vi "Histogram Bin Size Definition Dialog.vi"(8 "error in (no error)":errorcluster, 9 "Dialog? (T)":bool=TRUE, 11 "Histogram Options in":T1={"Bin Size"=nan, "Min Value"=nan, "Max Value"=nan, "Filter NaN & Infinite Values"=FALSE, "Frequency Plot"=FALSE, "Align Bins"=FALSE, "Bin Location"=enum."Left", "Project Outside Values"=FALSE, "Max Histogram Size"=-1} {"Max Histogram Size" format="%.0e"}) -> (0 "error out":errorcluster, 1 "Cancelled?":bool, 3 "Histogram Options":T1={"Bin Size"=1.0, "Min Value"=1.0, "Max Value"=1.0, "Filter NaN & Infinite Values"=FALSE, "Frequency Plot"=FALSE, "Align Bins"=FALSE, "Bin Location"=enum."Left", "Project Outside Values"=FALSE, "Max Histogram Size"=1} {"Max Histogram Size" format="%.0e"})   [LabVIEW 2019, in "Histogram Window.lvlib"]
doc: "Displays a standard dialog box that prompts users to enter information, such as a user name and password.\n--------------------\n\nThis Express VI is configured as follows:\n\nMessage to Display to the User:Histogram bin to use:\nThe inputs are: \nNumber: Bin"
uses:
  Histogram Window.lvlib
  Linear Histogram Options.ctl
  Histogram Bin Position.ctl
panel:
  in  "Histogram Options":T1={"Bin Size"=nan, "Min Value"=-inf, "Max Value"=inf, "Filter NaN & Infinite Values"=TRUE, "Frequency Plot"=FALSE, "Align Bins"=FALSE, "Bin Location"=enum."Left", "Project Outside Values"=FALSE, "Max Histogram Size"=100000} {"Max Histogram Size" format="%.0e"}
  in  "Cancel":bool
  in  "OK":bool caption="OK1"
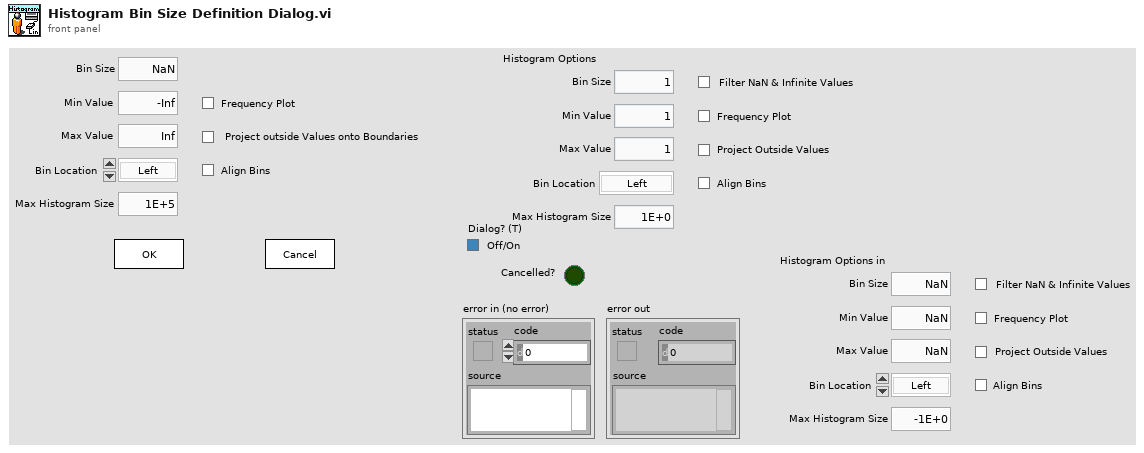
[diagram p1: front panel]
types:
  T1 = typedef "Linear Histogram Options.ctl" = cluster{"Bin Size":dbl, "Min Value":dbl, "Max Value":dbl, "Filter NaN & Infinite Values":bool, "Frequency Plot":bool, "Align Bins":bool, "Bin Location":T2, "Project Outside Values":bool, "Max Histogram Size":i32}
  T2 = typedef "Histogram Bin Position.ctl" = enum16{"Left", "Center", "Right"}
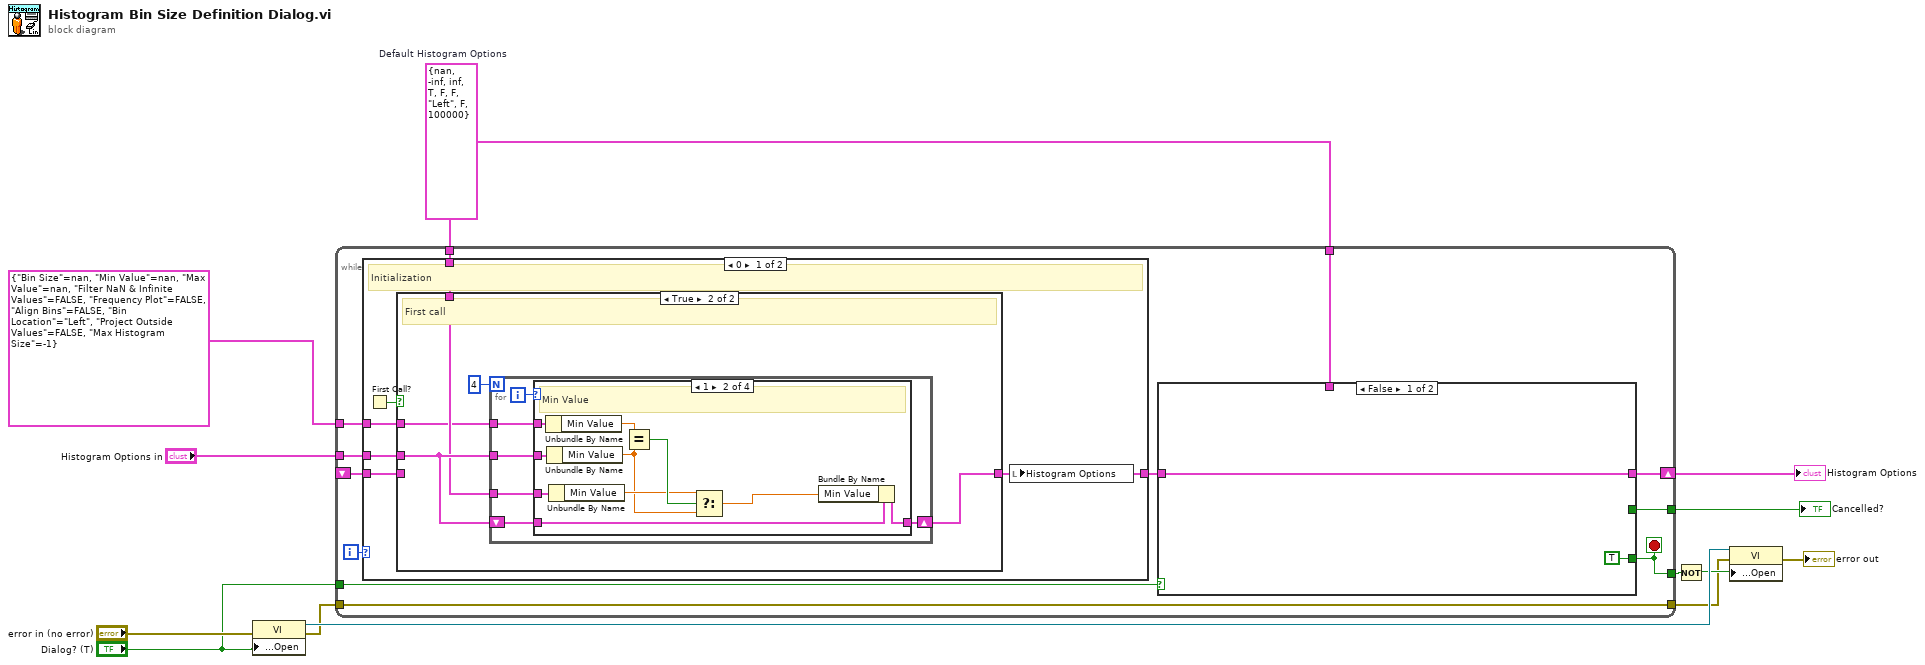
[diagram p0: block diagram]
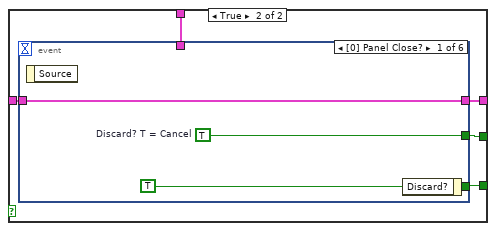
[diagram p2: hidden frame]
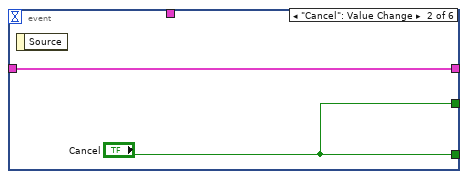
[diagram p3: hidden frame]
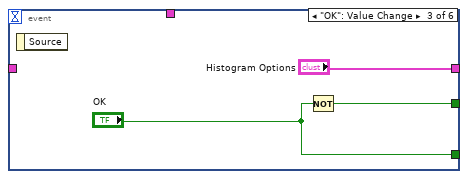
[diagram p4: hidden frame]
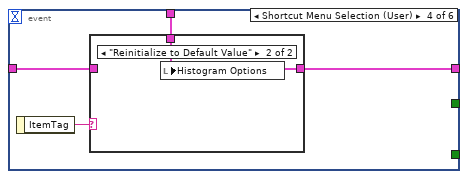
[diagram p5: hidden frame]
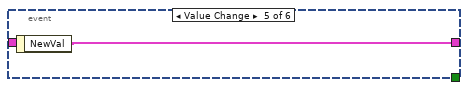
[diagram p7: hidden frame]
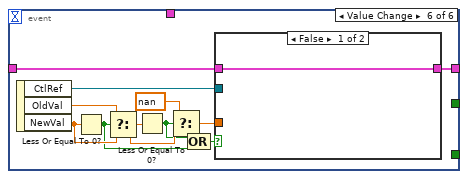
[diagram p8: hidden frame]
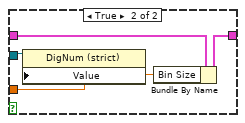
[diagram p9: hidden frame]
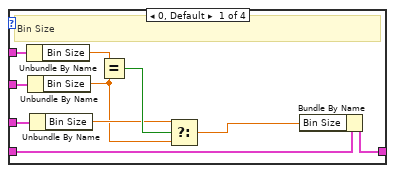
[diagram p11: hidden frame]
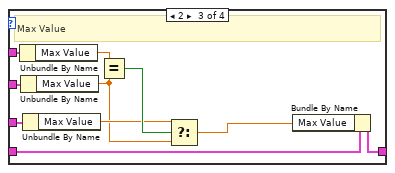
[diagram p12: hidden frame]
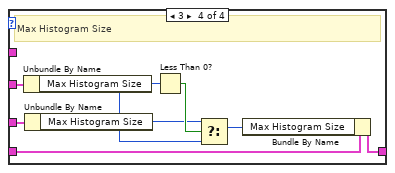
[diagram p13: hidden frame]
diagram:
  w6 = T1 {"Bin Size"=nan, "Min Value"=-inf, "Max Value"=inf, "Filter NaN & Infinite Values"=TRUE, "Frequency Plot"=FALSE, "Align Bins"=FALSE, "Bin Location"=enum."Left", "Project Outside Values"=FALSE, "Max Histogram Size"=100000}  # Default Histogram Options
  n1 = property class="VI"(error in="error in (no error)", "Front Panel Window:Open"="Dialog? (T)") -> (reference out=w10:refnum<vi>, error out=w5:errorcluster)  [unwired: 1 in]
  n2 = while {
    tunnel: [w25] -> w11
    tunnel: [w24] -> w9
    shift-right: [w23] -> w7
    shift-left: _ -> [w21]
    tunnel: w6 -> [w19]
    tunnel: w6 -> [w18]
    tunnel: "Histogram Options in" -> [w17]
    tunnel: w5 -> [w16]
    tunnel: [w16] -> w4
    tunnel: T1 {"Bin Size"=nan, "Min Value"=nan, "Max Value"=nan, "Filter NaN & Infinite Values"=FALSE, "Frequency Plot"=FALSE, "Align Bins"=FALSE, "Bin Location"=enum."Left", "Project Outside Values"=FALSE, "Max Histogram Size"=-1} ("Histogram Options in") -> [w15]
    tunnel: "Dialog? (T)" -> [w14]
    i -> [w22]
    stop <- w24 stop-if-true
    n3 = case "Initialization" shown="0" w22 {
      tunnel: w21 -> [w66 w120]
      tunnel: [w69 w120] -> w20
      tunnel: w19 -> [w65 _]
      tunnel: w17 -> [w68 _]
      tunnel: w15 -> [w64 _]
      frame 0 {
        # "Initialization"
        n4 = First Call?() -> (First Call?: T/F=w67:bool)
        n5 = case shown="True" w67 {
          tunnel: [w70 w75] -> w69
          tunnel: w68 -> [_ w74]
          tunnel: w66 -> [w70 _]
          tunnel: w65 -> [_ w73]
          tunnel: w64 -> [_ w72]
          frame False {
            # "Not first call: use previous values unless some valid options are provided"
          }
          frame True {
            # "First call"
            n6 = for {
              N: 4 -> [_]
              tunnel: w74 -> [w80]
              tunnel: w72 -> [w79]
              shift-right: [w77] -> w75
              shift-left: w74 -> [w78]
              tunnel: w73 -> [w76]
              i -> [w81]
              n7 = case shown="1" w81 {
                tunnel: w80 -> [w91 w101 w111 w119]
                tunnel: w79 -> [w90 w100 w110 _]
                tunnel: w78 -> [w85 w95 w105 w115]
                tunnel: [w83 w93 w103 w113] -> w77
                tunnel: w76 -> [w82 w92 w102 w112]
                frame 0, Default {
                  # "Bin Size"
                  n8 = Unbundle By Name(w90) -> ("Bin Size"=w89:dbl)
                  n9 = Unbundle By Name(w91) -> ("Bin Size"=w86:dbl)
                  n10 = Unbundle By Name(w82) -> ("Bin Size"=w87:dbl)
                  n11 = Equal?(x=w89, y=w86) -> (x = y?=w88:bool)
                  n12 = Select(t=w87, s=w88, f=w86) -> (s? t:f=w84:dbl)
                  n13 = Bundle By Name(cluster=w85, "Bin Size"=w84) -> (w83:T1)
                }
                frame 1 {
                  # "Min Value"
                  n14 = Unbundle By Name(w100) -> ("Min Value"=w99:dbl)
                  n15 = Unbundle By Name(w101) -> ("Min Value"=w96:dbl)
                  n16 = Unbundle By Name(w92) -> ("Min Value"=w97:dbl)
                  n17 = Equal?(x=w99, y=w96) -> (x = y?=w98:bool)
                  n18 = Select(t=w97, s=w98, f=w96) -> (s? t:f=w94:dbl)
                  n19 = Bundle By Name(cluster=w95, "Min Value"=w94) -> (w93:T1)
                }
                frame 2 {
                  # "Max Value"
                  n20 = Unbundle By Name(w110) -> ("Max Value"=w109:dbl)
                  n21 = Unbundle By Name(w111) -> ("Max Value"=w106:dbl)
                  n22 = Unbundle By Name(w102) -> ("Max Value"=w107:dbl)
                  n23 = Equal?(x=w109, y=w106) -> (x = y?=w108:bool)
                  n24 = Select(t=w107, s=w108, f=w106) -> (s? t:f=w104:dbl)
                  n25 = Bundle By Name(cluster=w105, "Max Value"=w104) -> (w103:T1)
                }
                frame 3 {
                  # "Max Histogram Size"
                  n26 = Unbundle By Name(w119) -> ("Max Histogram Size"=w116:i32)
                  n27 = Unbundle By Name(w112) -> ("Max Histogram Size"=w117:i32)
                  n28 = Less Than 0?(x=w116) -> (x < 0?=w118:bool)
                  n29 = Select(t=w117, s=w118, f=w116) -> (s? t:f=w114:i32)
                  n30 = Bundle By Name(cluster=w115, "Max Histogram Size"=w114) -> (w113:T1)
                }
              }
            }
          }
        }
        n31 = local write "Histogram Options"(w69) -> ()
      }
      frame 1, Default {
        # "user interaction"
      }
    }
    n32 = case shown="False" w14 {
      tunnel: [_ w32] -> w25
      tunnel: [TRUE ("OK") w31] -> w24
      tunnel: [w27 w30] -> w23
      tunnel: w20 -> [w27 w29]
      tunnel: w18 -> [_ w28]
      frame False {
      }
      frame True {
        n33 = event shown="[0] Panel Close?" {
          selector: _ -> [_ _ _ _ _ _]
          dyn-events: _ -> [_ _ _ _ _ _]
          timeout: _ -> [_ _ _ _ _ _]
          tunnel: [w35 "Cancel" "OK" _ _ _] -> w31
          tunnel: [w34 "Cancel" w38 _ _ _] -> w32
          tunnel: [w33 w37 "Histogram Options" w42 w47 w48] -> w30
          tunnel: w29 -> [w33 w37 _ w43 _ w49]
          tunnel: w28 -> [_ _ _ w41 _ _]
          event Panel Close? {
            w34 = TRUE  # Discard? T = Cancel
            w35 = TRUE ("Discard?")
            n34 = event-data() -> ()  [unwired: 1 in, 1 out]
            n35 = event-data("Discard?"=w35) -> ()  [unwired: 1 in, 1 out]
          }
          event "Cancel": Value Change {
            n36 = event-data() -> ()  [unwired: 1 in, 1 out]
          }
          event "OK": Value Change {
            n37 = event-data() -> ()  [unwired: 1 in, 1 out]
            n38 = Not(x="OK") -> (.not. x?=w38:bool)
          }
          event Shortcut Menu Selection (User) {
            n39 = event-data() -> ("ItemTag"=w44:string)  [unwired: 1 in]
            n40 = case shown="\"Reinitialize to Default Value\"" w44 {
              tunnel: w43 -> [w45 _]
              tunnel: [w45 w46] -> w42
              tunnel: w41 -> [_ w46]
              frame "", Default {
              }
              frame "Reinitialize to Default Value" {
                n41 = local write "Histogram Options"(w46) -> ()
              }
            }
          }
          event Value Change {
            n42 = event-data() -> ("NewVal"=w47:T1)  [unwired: 1 in]
          }
          event Value Change {
            n43 = event-data() -> ("CtlRef"=w51:refnum<vi>, "OldVal"=w57:dbl, "NewVal"=w58:dbl)  [unwired: 1 in]
            n44 = Less Or Equal To 0?(x=w58) -> (x <= 0?=w52:bool)
            n45 = Select(t=w57, s=w52, f=w58) -> (s? t:f=w56:dbl)
            n46 = Less Or Equal To 0?(x=w56) -> (x <= 0?=w54:bool)
            n47 = Select(t=nan, s=w54, f=w56) -> (s? t:f=w50:dbl)
            n48 = Compound Arithmetic op=OR(w54, w52) -> (w53:bool)
            n49 = case shown="False" w53 {
              tunnel: w51 -> [_ w63]
              tunnel: w50 -> [_ w61]
              tunnel: w49 -> [w59 w62]
              tunnel: [w59 w60] -> w48
              frame False {
              }
              frame True {
                n50 = property class="DigNum (strict)"(reference=w63, "Value"=w61) -> ()  [unwired: 1 in, 2 out]
                n51 = Bundle By Name(cluster=w62, "Bin Size"=w61) -> (w60:T1)
              }
            }
          }
        }
      }
    }
  }
  "Cancelled?" <- w11
  "Histogram Options" <- w7
  n52 = Not(x=w9) -> (.not. x?=w8:bool)
  n53 = property class="VI"(reference=w10, error in=w4, "Front Panel Window:Open"=w8) -> (error out=→"error out":errorcluster)  [unwired: 1 out]
